vi "Day11-update_around_flash.vi"(9 "Flash Location":cluster{i32, i32}, 11 "Energy Levels":i32[][](array[numeric])) -> (3 "Energy Levels out":i32[][](array[numeric]))   [LabVIEW 2021]
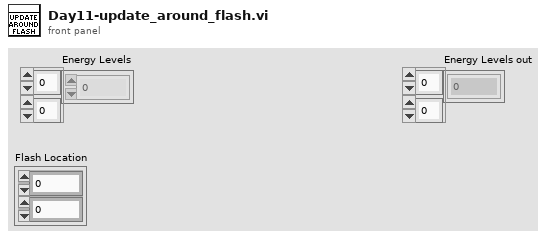
[diagram p1: front panel]
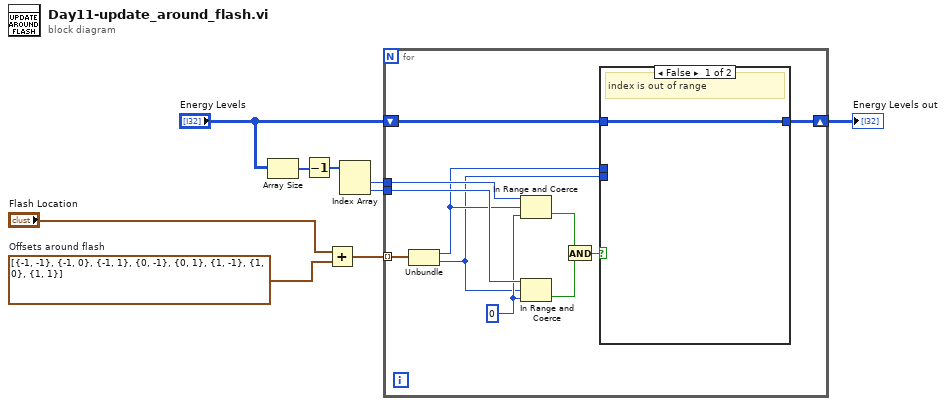
[diagram p0: block diagram]
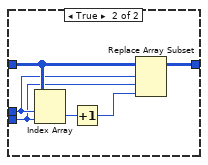
[diagram p2: hidden frame]
diagram:
  w8 = cluster{i32, i32}[] [{-1, -1}, {-1, 0}, {-1, 1}, {0, -1}, {0, 1}, {1, -1}, {1, 0}, {1, 1}]  # Offsets around flash
  n1 = Array Size(array="Energy Levels") -> (size(s)=w4:i32[])
  n2 = Decrement(x=w4) -> (x-1=w3:i32[])
  n3 = Add(x="Flash Location", y=w8) -> (x+y=w7:cluster{i32, i32}[])
  n4 = Index Array(array=w3) -> (element #1=w2:i32, element #2=w1:i32)  [unwired: 2 in]
  n5 = for {
    tunnel: w7 -> [w20] mode=indexing
    shift-right: [w10] -> w6
    shift-left: "Energy Levels" -> [w11]
    tunnel: w2 -> [w19]
    tunnel: w1 -> [w18]
    w17 = 0 ("lower limit")
    n6 = Unbundle(w20) -> (w13:i32, w12:i32)
    n7 = In Range and Coerce(upper limit=w19, x=w13, lower limit=w17) -> (In Range?=w15:bool)  [unwired: 1 out]
    n8 = In Range and Coerce(upper limit=w18, x=w12, lower limit=w17) -> (In Range?=w16:bool)  [unwired: 1 out]
    n9 = And(x=w15, y=w16) -> (x .and. y?=w14:bool)
    n10 = case shown="False" w14 {
      tunnel: w11 -> [w21 w26]
      tunnel: w13 -> [_ w23]
      tunnel: w12 -> [_ w22]
      tunnel: [w21 w25] -> w10
      frame False {
        # "index is out of range"
      }
      frame True {
        n11 = Index Array(array=w26, index (row)=w23, index (col)=w22) -> (element=w27:i32)
        n12 = Increment(x=w27) -> (x+1=w24:i32)
        n13 = Replace Array Subset(array=w26, new element=w24, index (row)=w23, index (col)=w22) -> (w25:i32[][])
      }
    }
  }
  "Energy Levels out" <- w6
